vi "VFH-compare_data.vi"() -> ()   [LabVIEW 2020, in "VFH-VNA_File_Handler.lvlib"]
uses:
  VFH-VNA_File_Handler.lvlib
panel:
  out "XY Graph 2":cluster{"Frequency":dbl[], "S11_Imag":dbl[]}[](graph)
  out "real":cluster{"Frequency":dbl[], "S11_Real":dbl[]}[](graph)
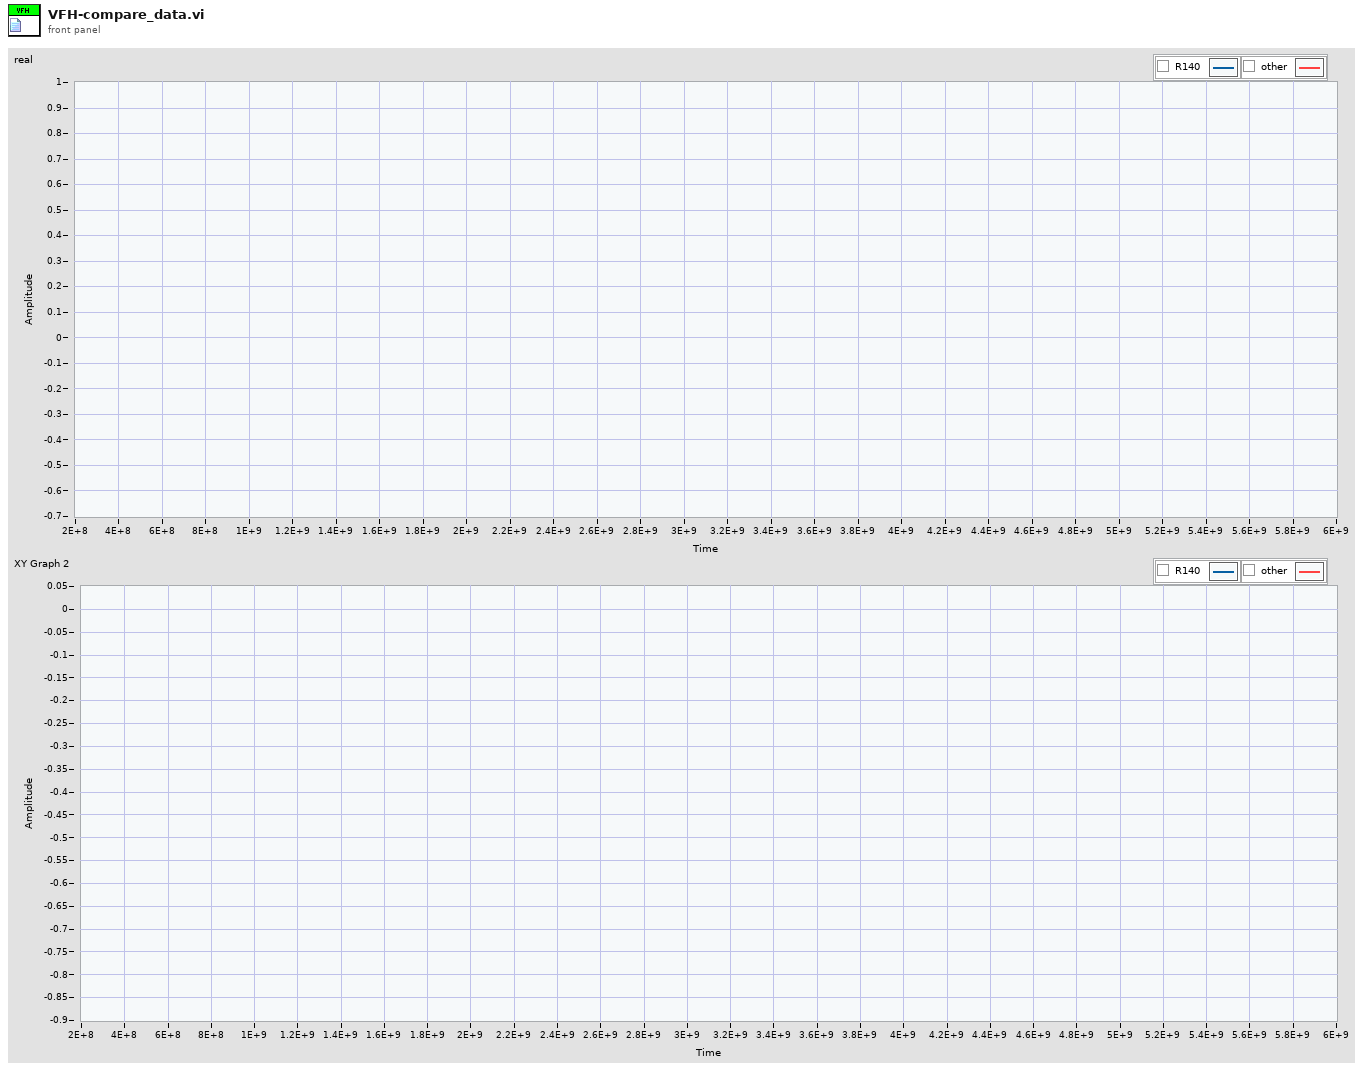
[diagram p1: front panel]
types:
  T1 = typedef "VFH-VNA_File_Handler.lvlib/VFH-file_cluster-r140.ctl" = cluster{"Frequency":dbl[], "Permativity'":dbl[], "Permativity''":dbl[], "Q [S/m]":dbl[], "Tan":dbl[], "Reflection R":dbl[], "Reflection I":dbl[]}
  T2 = typedef "VFH-VNA_File_Handler.lvlib/VFH-file_cluster-NanoVNA.ctl" = cluster{"Frequency":dbl[], "S11_Real":dbl[], "S11_Imag":dbl[], "S21_Real":dbl[], "S21_Imag":dbl[], "S12_Real":dbl[], "S12_Imag":dbl[], "S22_Real":dbl[], "S22_Imag":dbl[]}
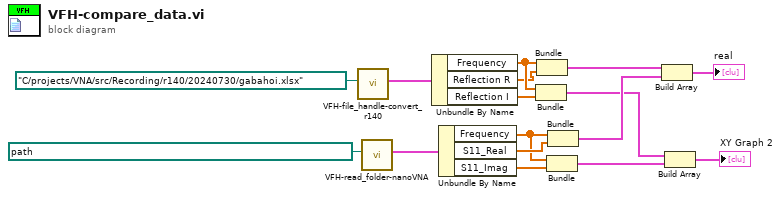
[diagram p0: block diagram]
diagram:
  n1 = call "VFH-file_handle-convert_r140.vi"("file path (dialog if empty)"=path "C:/projects/VNA/src/Recording/r140/20240730/gabahoi.xlsx") -> ("Handled data"=w14:T1)  [unwired: 10 in]
  n2 = call "VFH-read_folder-nanoVNA.vi"("Folder Path"=path "C:/projects/VNA/src/Recording/minivna/Test-gabahøy/record") -> ("avg output"=w13:T2)  [unwired: 7 in, 3 out]
  n3 = Unbundle By Name(w14) -> ("Frequency"=w9:dbl[], "Reflection R"=w8:dbl[], "Reflection I"=w7:dbl[])
  n4 = Unbundle By Name(w13) -> ("Frequency"=w11:dbl[], "S11_Real"=w12:dbl[], "S11_Imag"=w10:dbl[])
  n5 = Bundle("Frequency"=w9, "Reflection I"=w7) -> (w3:cluster{"Frequency":dbl[], "Reflection I":dbl[]})  [unwired: 1 in]
  n6 = Bundle("Frequency"=w9, "Reflection R"=w8) -> (w6:cluster{"Frequency":dbl[], "Reflection R":dbl[]})  [unwired: 1 in]
  n7 = Bundle("Frequency"=w11, "S11_Imag"=w10) -> (w4:cluster{"Frequency":dbl[], "S11_Imag":dbl[]})  [unwired: 1 in]
  n8 = Bundle("Frequency"=w11, "S11_Real"=w12) -> (w5:cluster{"Frequency":dbl[], "S11_Real":dbl[]})  [unwired: 1 in]
  n9 = Build Array(w6, w5) -> (→"real":cluster{"Frequency":dbl[], "S11_Real":dbl[]}[])
  n10 = Build Array(w3, w4) -> (→"XY Graph 2":cluster{"Frequency":dbl[], "S11_Imag":dbl[]}[])
